vi "Write meas.ready.vi"(10 "meas.ready":bool, 11 "sync.resources":T1) -> (3 "sync.resources":T1)   [LabVIEW 2013, in "ni579x Synchronization v1 FPGA.lvlib"]
uses:
  <instrlib>/ni579x/Synchronization/v1/FPGA/ni579x Synchronization v1 FPGA.lvlib
  <instrlib>/ni579x/Synchronization/v1/FPGA/Implementation/Resources.ctl
  <vilib>/rvi/DataTransferAndStorage/Container/Common/niFpgaContainerExecOnDevCompGetState.vi
  <vilib>/rvi/DataTransferAndStorage/Register/Emulation/niFpgaRegisterEmulationFpgaImpl.vi
  <instcachedir>/0/niFpgaRegisterEmulationFpgaImpl_DCF4BC0110594B98B44A971D60CEEC4D.lvgen/niFpgaRegisterEmulationFpgaImpl_DCF4BC0110594B98B44A971D60CEEC4D_002.vi
  <vilib>/rvi/DataTransferAndStorage/Container/Common/niFpgaContainerGetUniqueNameForEmu.vi
  <vilib>/rvi/DataTransferAndStorage/Container/XNode/niFpgaContainer.xnode
  <vilib>/rvi/DataTransferAndStorage/Register/Emulation/niFpgaRegisterEmulationRefIn.vi
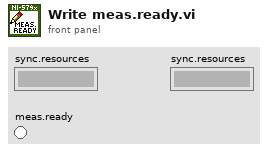
[diagram p1: front panel]
types:
  T1 = typedef "ni579x Synchronization v1 FPGA.lvlib/Resources.ctl" = cluster{"master":refnum<k21>, "meas.enable":refnum<k21>, "meas.ready":refnum<k21>, "meas.arm":refnum<k21>, "meas.valid":refnum<k21>, "meas.value":refnum<k21>, "meas.oversample clock":refnum<k21>, "meas.oversample factor":refnum<k21>, "cptr":refnum<k21>, "cptr.adjust":refnum<k21>, "cptr.period":refnum<k21>}
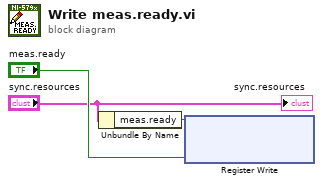
[diagram p0: block diagram]
diagram:
  n1 = Unbundle By Name("sync.resources") -> ("meas.ready"=w3:refnum<k21>)
  n2 = xnode ("Register Write")("Data"="meas.ready", "Register In"=w3) -> ()  [unwired: 1 out]
  "sync.resources" <- "sync.resources"
